vi "Get All Subaddress and Mode Codes in Remote Terminal.vi"(8 "error in":errorcluster, 11 "remote terminal":T1 format="%.0x") -> (0 "error out":errorcluster, 2 "subaddress sections":T1[](array[typedef]) format="%.0x", 3 "remote terminal out":T1 format="%.0x")   [LabVIEW 2020, in "AIM MIL-STD-1553 Scripting.lvlib"]
doc: "Returns all of the <b>subaddress sections</b> in the <b>remote terminal</b>."
uses:
  AIM MIL-STD-1553 Scripting.lvlib
  <vilib>/NI VeriStand/Custom Device Tools/Custom Device Utility Library/Custom Device Utility Library.lvlib
  Constants.vi
  <vilib>/NI VeriStand/Custom Device Tools/Custom Device Utility Library/NI VeriStand - Search for All Items by GUID.vi
  <vilib>/NI VeriStand/Custom Device API/Custom Device Item Ref.ctl
  <vilib>/NI VeriStand/Custom Device API/Custom Device API.lvlib
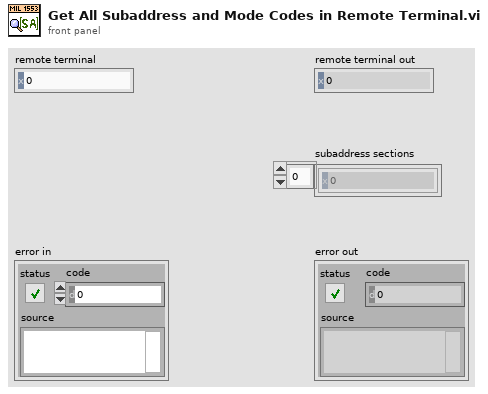
[diagram p1: front panel]
types:
  T1 = typedef "Custom Device API.lvlib/Custom Device Item Ref.ctl" = u64
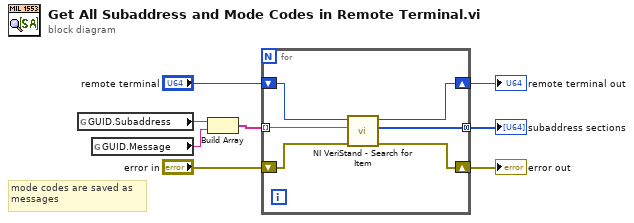
[diagram p0: block diagram]
diagram:
  # "mode codes are saved as \nmessages"
  n1 = global read "Constants.vi" "GUID.Subaddress"() -> (w2:string)
  n2 = global read "Constants.vi" "GUID.Message"() -> (w1:string)
  n3 = Build Array(w2, w1) -> (w3:string[])
  n4 = for {
    tunnel: w3 -> [w14] mode=indexing
    tunnel: [w9] -> w4 mode=concatenating
    shift-right: [w10] -> w5
    shift-left: "error in" -> [w13]
    shift-right: [w11] -> w6
    shift-left: "remote terminal" -> [w12]
    n5 = call-poly <vilib>:"NI VeriStand - Search for Item.vi"("error in"=w13, "Item GUID"=w14, "Section Ref in"=w12) -> ("error out"=w10:errorcluster, "Item Refs"=w9:T1[], "Section Ref out"=w11:T1)  [unwired: 5 in, 1 out]
  }
  "remote terminal out" <- w6
  "error out" <- w5
  "subaddress sections" <- w4
